vi "Design Challenge _ HW2 V2.vi"() -> ()   [LabVIEW 2025]
uses:
  <vilib>/numeric/Random Number (Range) DBL.vi
panel:
  out "XY Graph":cluster{"Y":dbl[], "Y":dbl[]}[](graph)
  out "X":dbl
  out "Height - Y":dbl
  in  "Initial Height":dbl
  in  "Initial Velocity":dbl
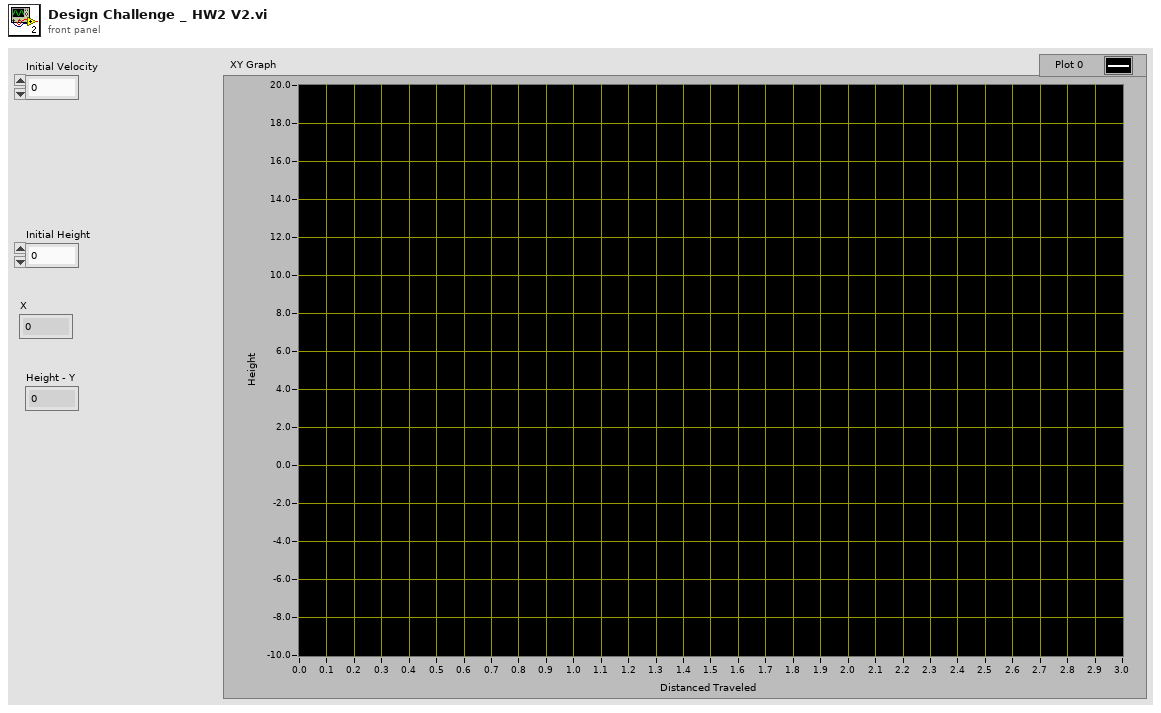
[diagram p1: front panel]
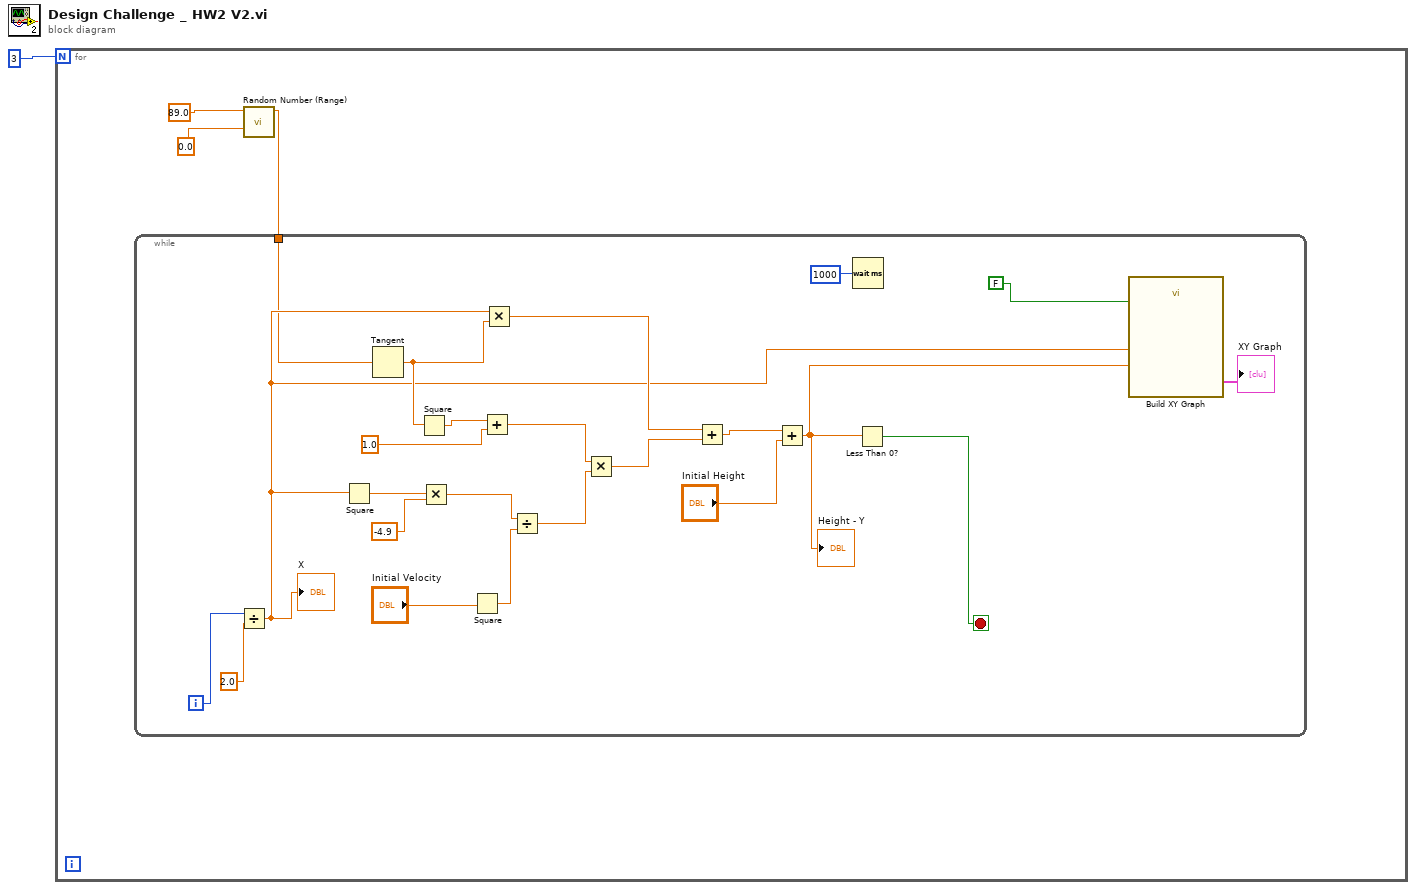
[diagram p0: block diagram]
diagram:
  n1 = for {
    N: 3 -> [_]
    n2 = call-poly <vilib>:"Random Number (Range).vi"("lower bound (0)"=0.0, "upper bound (100)"=89.0) -> ("number"=w4:dbl)  [unwired: 9 in]
    n3 = while {
      tunnel: w4 -> [w5]
      i -> [w27]
      stop <- w11 stop-if-true
      n4 = Divide(x=w27, y=2.0) -> (x/y=w8:dbl)
      "X" <- w8
      n5 = Square(x=w8) -> (x^2=w22:dbl)
      n6 = Tangent(1:w5) -> (0:w25:dbl)
      n7 = Square(x=w25) -> (x^2=w23:dbl)
      n8 = Multiply(x=w22, y=-4.9) -> (x*y=w19:dbl)
      n9 = Square(x="Initial Velocity") -> (x^2=w18:dbl)
      n10 = Add(x=w23, y=1.0) -> (x+y=w17:dbl)
      n11 = Multiply(x=w8, y=w25) -> (x*y=w15:dbl)
      n12 = Divide(x=w19, y=w18) -> (x/y=w16:dbl)
      n13 = Multiply(x=w17, y=w16) -> (x*y=w14:dbl)
      n14 = Add(x=w15, y=w14) -> (x+y=w12:dbl)
      n15 = Add(x=w12, y="Initial Height") -> (x+y=w9:dbl)
      "Height - Y" <- w9
      n16 = Wait (ms)(milliseconds to wait=u32 1000 ("millisecond timer value")) -> ()  [unwired: 1 out]
      n17 = Less Than 0?(x=w9) -> (x < 0?=w11:bool)
      n18 = call "Build XY Graph"("Reset"=FALSE, "Y Input"=w9, "X Input"=w8) -> ("XY Graph"=→"XY Graph":cluster{"X":dbl[], "Y":dbl[]}[])  [unwired: 7 in, 1 out]
    }
  }
